vi "LED Color.vi"(11 "Result":bool) -> (3 "s? t:f":cluster{u32, u32}[](array[cluster]))   [LabVIEW 2021]
panel:
  out "Colors [4]":cluster{u32, u32}[](array[cluster])
  out "Boolean":bool
  in  "Blank Button":bool
  out "Red":cluster{u32, u32}[](array[cluster])
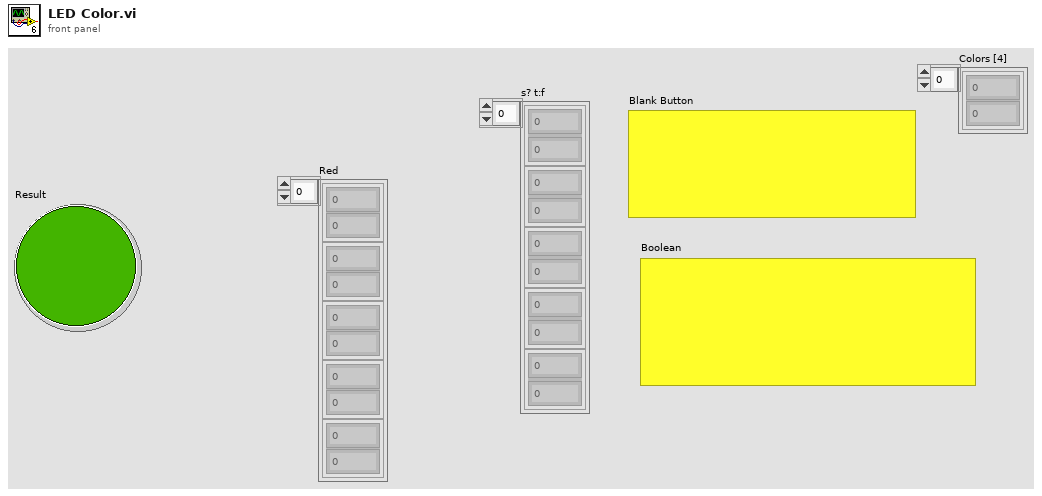
[diagram p1: front panel]
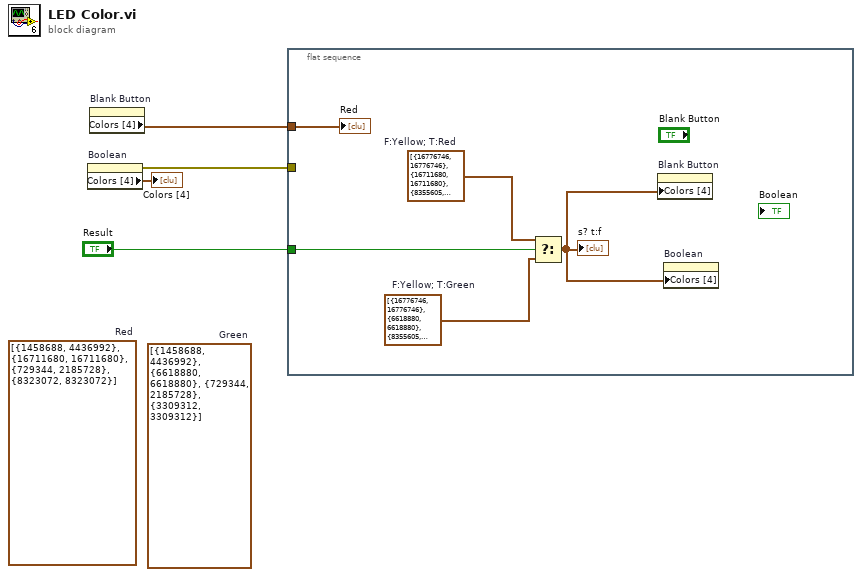
[diagram p0: block diagram]
diagram:
  (unwired) cluster{u32, u32}[] [{1458688, 4436992}, {6618880, 6618880}, {729344, 2185728}, {3309312, 3309312}]  # Green
  (unwired) cluster{u32, u32}[] [{1458688, 4436992}, {16711680, 16711680}, {729344, 2185728}, {8323072, 8323072}]  # Red
  n1 = property on="Boolean" class="Bool (strict)"() -> (error out=w1:errorcluster, "Colors [4]"=→"Colors [4]":cluster{u32, u32}[])  [unwired: 2 in, 1 out]
  n2 = property on="Blank Button" class="Bool"() -> ("Colors [4]"=w4:cluster{u32, u32}[])  [unwired: 2 in, 2 out]
  n3 = flat-sequence {
    tunnel: w4 -> [w9]
    tunnel: "Result" -> [w8]
    tunnel: w1 -> [_]
    frame #0 {
      w7 = cluster{u32, u32}[] [{16776746, 16776746}, {16711680, 16711680}, {8355605, 8355605}, {8323072, 8323072}]  # F:Yellow; T:Red
      w6 = cluster{u32, u32}[] [{16776746, 16776746}, {6618880, 6618880}, {8355605, 8355605}, {3309312, 3309312}]  # F:Yellow; T:Green
      n4 = Select(t=w7, s=w8, f=w6) -> (s? t:f=w5:cluster{u32, u32}[])
      "s? t:f" <- w5
      n5 = property on="Blank Button" class="Bool"("Colors [4]"=w5) -> ()  [unwired: 2 in, 2 out]
      n6 = property on="Boolean" class="Bool (strict)"("Colors [4]"=w5) -> ()  [unwired: 2 in, 2 out]
      "Red" <- w9
    }
  }
